vi "Group GUID.vi"() -> (3 "GUID":string="88fcfa75-3196-4ae9-a459-f2e46a72afc7")   [LabVIEW 2017, in "Data Sharing Framework System Explorer.lvlib"]
uses:
  Data Sharing Framework System Explorer.lvlib
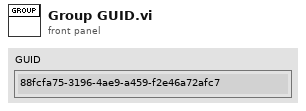
[diagram p1: front panel]
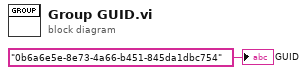
[diagram p0: block diagram]
diagram:
  "GUID" <- "0b6a6e5e-8e73-4a66-b451-845da1dbc754" ("Data Sharing Framework")
